vi "thermalImage_main02.vi"() -> ()   [LabVIEW 2018]
doc: "This example performs writes and reads on a serial port, as directed by the user. You can press the Write and Read buttons, and change the Read Count, while the example is running.\n\nThe parameters set for the serial port must match the parameters of the connected instrument or device. In this example, the Read Count parameter specifies the number of bytes that the serial port reads. If there were more bytes at the port than the specified number, those bytes would not be read. If there were less bytes at the port than the specified number, you would receive a timeout error.\n\nThis example expands upon the flow control options for XON and XOFF, allowing the user to choose those control characters. Also, the user can enable or disable a termination character. Some devices require a termination character in order to identify the end of command strings. Some devices send a termination character to signify the end of data to be read. This example shows how you can end the Read operation once a termination character is detected in the buffer and/or append a termination character at the end of the Write data."
uses:
  <vilib>/userdefined/High Color/IMAQdx.ctl
  <vilib>/Instr/_visa.llb/VISA Configure Serial Port (Instr).vi
  <vilib>/vision/driver/NI_Vision_Acquisition_Software.lvlib
  <vilib>/vision/NI_Vision_Development_Module.lvlib
panel:
  out "최대온도":dbl
  out "웨이브폼 차트":dbl(graph)
  in  "Frames Per Second":u32=10
  in  "AVI Path":path=path "E:/temp/b.avi"
  in  "stop 4":bool
  in  "stop 3":bool
  out "Cam  2":T1(plugin-control)
  in  "Camera":T2="cam1"
  in  "stop":bool
  in  "stop 2":bool
  in  "폭":dbl=10.0
  in  "중심":dbl=35.0
  out "Temperature":dbl[][](graph)
  in  "Stop":bool
  in  "VISA resource name":refnum<visa-resource-name>="COM6"
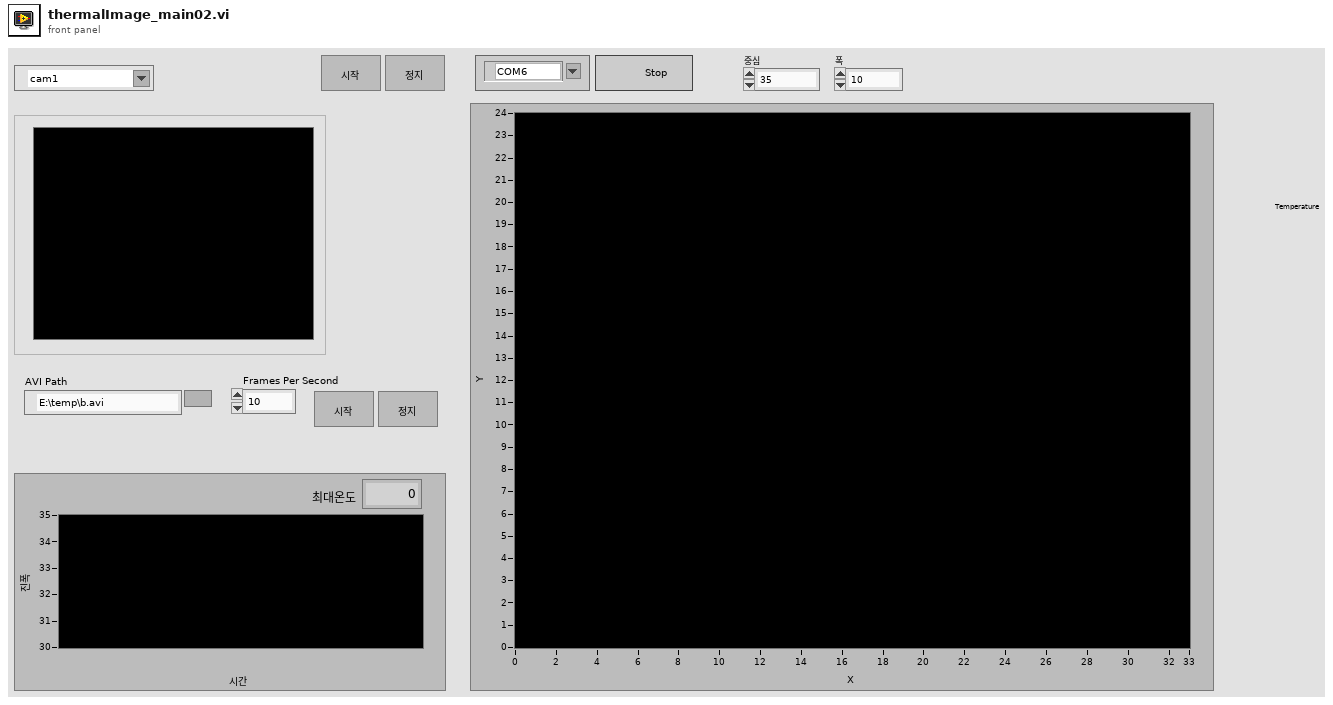
[diagram p1: front panel]
types:
  T1 = typedef "IMAQ Image.ctl" = refnum<image>
  T2 = typedef "IMAQdx.ctl" = refnum<k21>
  T3 = typedef "Image Type" = u32
  T4 = typedef "IMAQ AVI2 Refnum.ctl" = refnum<k20>
  T5 = typedef "imagedata.ctl" = cluster{"image type":i32, "image depth":i32, "image":u8[], "mask":u8[], "colors":u32[], "Rectangle":cluster{"left":i16, "top":i16, "right":i16, "bottom":i16}}
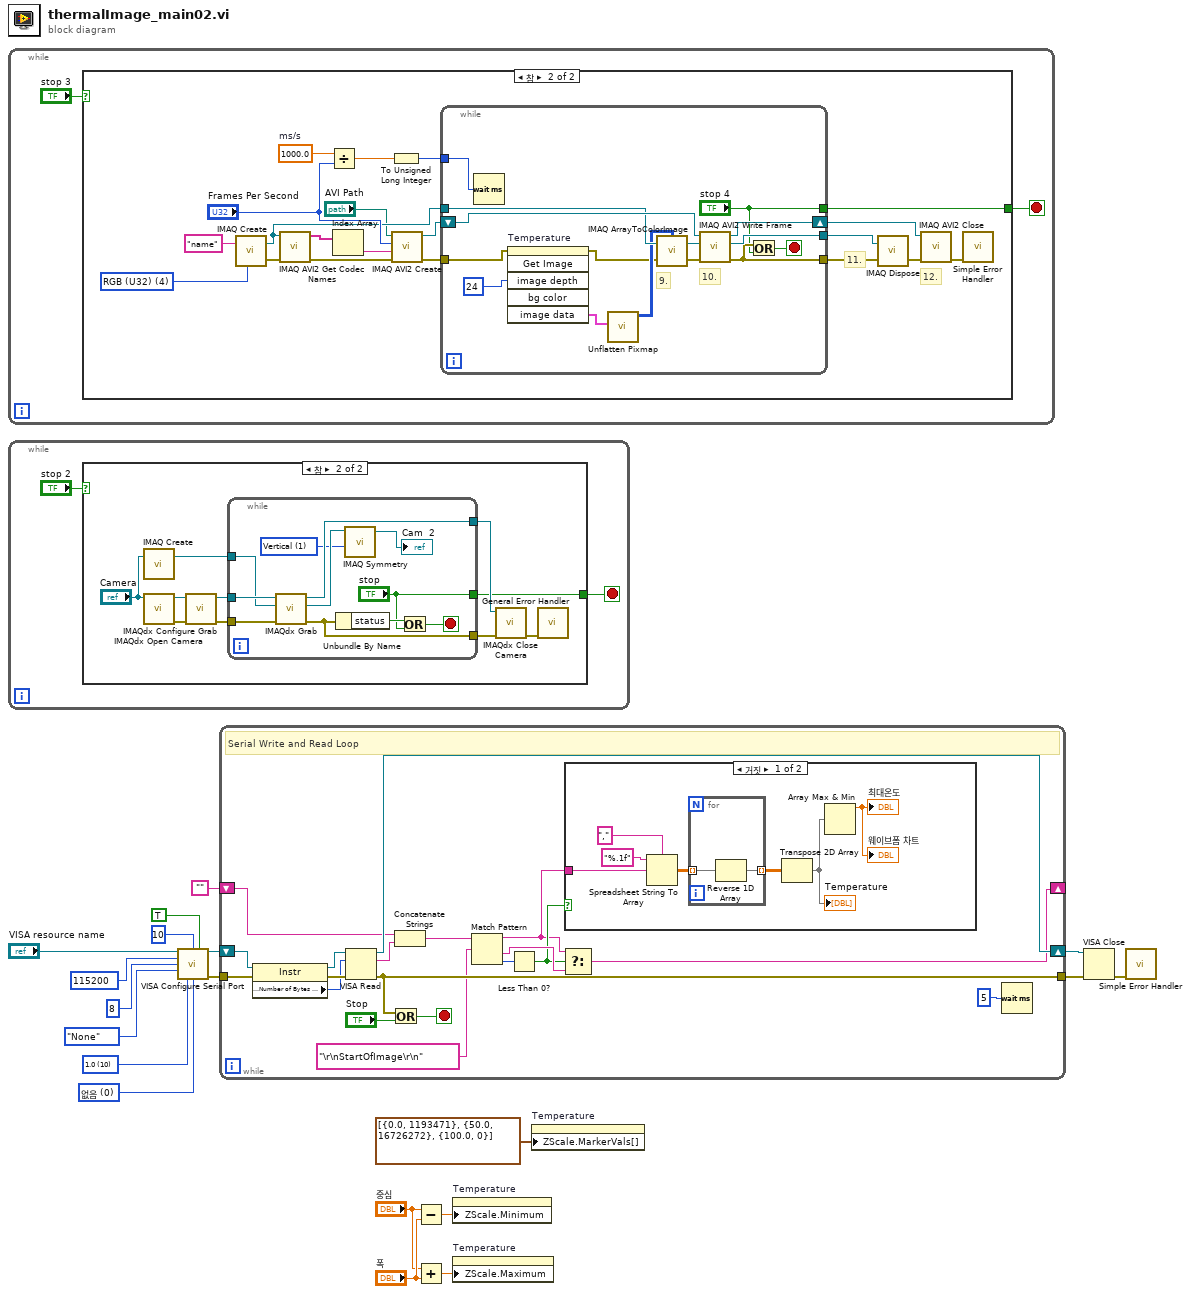
[diagram p0: block diagram]
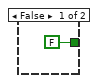
[diagram p2: hidden frame]
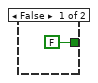
[diagram p3: hidden frame]
diagram:
  w6 = u16 0 items=["없음", "XON/XOFF", "RTS/CTS", "XON/XOFF & RTS/CTS", "DTR/DSR", "XON/XOFF & DTR/DSR"] ("flow control (0:none)")
  w7 = u16 10 items=["1.0"=10, "1.5"=15, "2.0"=20] ("stop bits (10: 1 bit)")
  n1 = while {
    stop <- w20 stop-if-true
    n2 = case shown="참" "stop 3" {
      tunnel: [FALSE ("stop") w23] -> w20
      frame False {
      }
      frame True {
        w26 = 1000.0  # ms/s
        w24 = T3 4 items=["Grayscale (U8)", "Grayscale (I16)", "Grayscale (SGL)", "Complex (CSG)", "RGB (U32)", "HSL (U32)", "RGB (U64)", "Grayscale (U16)"] ("Image Type")
        # "12."
        # "11."
        n3 = call "IMAQ Create"("Image Name"="name", "Image Type"=w24) -> ("New Image"=w36:T1, "error out"=w35:errorcluster)  [unwired: 3 in]
        n4 = call "IMAQ AVI2 Get Codec Names"("error in (no error)"=w35, "Image"=w36) -> ("error out"=w34:errorcluster, "Codec Names"=w38:string[])  [unwired: 8 in]
        n5 = Divide(x=w26, y="Frames Per Second") -> (x/y=w41:dbl)
        n6 = Index Array(array=w38) -> (element=w39:string)  [unwired: 1 in]
        n7 = To Unsigned Long Integer(number=w41) -> (unsigned 32bit integer=w42:u32)
        n8 = call "IMAQ AVI2 Create"("error in (no error)"=w34, "Codec"=w39, "Frames Per Second"="Frames Per Second", "AVI Path"="AVI Path") -> ("error out"=w37:errorcluster, "AVI Refnum"=w33:T4)  [unwired: 6 in]
        n9 = while {
          tunnel: w36 -> [w51]
          tunnel: w37 -> [w45]
          tunnel: [w55] -> w27
          tunnel: [w52] -> w28
          shift-right: [w56] -> w29
          shift-left: w33 -> [w57]
          tunnel: w42 -> [w54]
          tunnel: ["stop 4"] -> w23
          stop <- w53 stop-if-true
          # "10."
          # "9."
          n10 = Wait (ms)(milliseconds to wait=w54) -> ()  [unwired: 1 out]
          n11 = invoke on="Temperature" class="IntGraph (엄격한)" method="Get Image"(error in=w45, "image depth"=24 ("Image Depth")) -> (error out=w44:errorcluster, "image data"=w46:T5)  [unwired: 4 in, 4 out]
          n12 = call <vilib>:"Unflatten Pixmap.vi"("image data"=w46) -> ("24-bit pixmap"=w48:u32[][])  [unwired: 4 in, 6 out]
          n13 = call "IMAQ ArrayToColorImage"("Image Pixels (U32)"=w48, "Image"=w51, "error in (no error)"=w44) -> ("Image Out"=w50:T1, "error out"=w49:errorcluster)  [unwired: 2 in]
          n14 = call "IMAQ AVI2 Write Frame"("error in (no error)"=w49, "Image"=w50, "AVI Refnum"=w57) -> ("error out"=w52:errorcluster, "Image Out (duplicate)"=w55:T1, "AVI Refnum (duplicate)"=w56:T4)  [unwired: 6 in]
          n15 = Or(x=w52, y="stop 4") -> (x .or. y?=w53:bool)
        }
        n16 = call "IMAQ Dispose"("Image"=w27, "error in (no error)"=w28) -> ("error out"=w30:errorcluster)  [unwired: 4 in]
        n17 = call "IMAQ AVI2 Close"("error in (no error)"=w30, "AVI Refnum"=w29) -> ("error out"=w31:errorcluster)  [unwired: 9 in]
        n18 = call <vilib>:"Simple Error Handler.vi"("error in (no error)"=w31) -> ()  [unwired: 4 in, 5 out]
      }
    }
  }
  n19 = while {
    stop <- w58 stop-if-true
    n20 = case shown="참" "stop 2" {
      tunnel: [FALSE ("stop") w61] -> w58
      frame False {
      }
      frame True {
        n21 = call "IMAQ Create"("Image Name"="Camera") -> ("New Image"=w70:T1)  [unwired: 3 in, 2 out]
        n22 = call <vilib>:"IMAQdx Open Camera.vi"("Session In"="Camera") -> ("error out"=w64:errorcluster, "Session Out"=w66:T2)  [unwired: 2 in, 7 out]
        n23 = call <vilib>:"IMAQdx Configure Grab.vi"("error in"=w64, "Session In"=w66) -> ("error out"=w62:errorcluster, "Session Out"=w63:T2)  [unwired: 1 in, 7 out]
        n24 = while {
          tunnel: [w76] -> w69
          tunnel: w62 -> [w78]
          tunnel: w63 -> [w79]
          tunnel: [w75] -> w68
          tunnel: w70 -> [w77]
          tunnel: ["stop"] -> w61
          stop <- w81 stop-if-true
          w71 = u32 1 items=["Horizontal", "Vertical", "Central", "1st Diagonal", "2nd Diagonal"] ("Type of Symmetry")
          n25 = call <vilib>:"IMAQdx Grab.vi"("error in"=w78, "Image In"=w77, "Session In"=w79) -> ("error out"=w75:errorcluster, "Image Out"=w73:T1, "Session Out"=w76:T2)  [unwired: 5 in, 1 out]
          n26 = Unbundle By Name(w75) -> ("status"=w80:bool)
          n27 = call "IMAQ Symmetry"("Type of Symmetry"=w71, "Image Src"=w73) -> ("Image Dst Out"=→"Cam  2":T1)  [unwired: 3 in, 1 out]
          n28 = Or(x=w80, y="stop") -> (x .or. y?=w81:bool)
        }
        n29 = call <vilib>:"IMAQdx Close Camera.vi"("error in"=w68, "Session In"=w69) -> ("error out"=w67:errorcluster)  [unwired: 9 out]
        n30 = call <vilib>:"General Error Handler.vi"("error in (no error)"=w67) -> ()  [unwired: 2 in, 13 out]
      }
    }
  }
  n31 = call-poly "VISA Configure Serial Port"("VISA resource name"="VISA resource name", "termination char\n(0xA = '\\n' = LF)"=u8 10 ("Termination Character"), "Enable Termination\nChar (T)"=TRUE ("End Read on Termination Character?"), "baud rate (9600)"=u32 115200, "data bits (8)"=u16 8, "parity (0:none)"=enum16{"None", "Odd", "Even", "Mark", "Space"}."None", "stop bits (10: 1 bit)"=w7, "flow control (0:none)"=w6) -> ("VISA resource name out"=w13:refnum<visa-resource-name>, "error out"=w12:errorcluster)  [unwired: 2 in, 4 out]
  n32 = while {
    shift-right: [w95] -> w15
    shift-left: w13 -> [w97]
    tunnel: w12 -> [w93]
    tunnel: [w89] -> w16
    shift-right: [w82] -> _
    shift-left: "" -> [w91]
    stop <- w99 stop-if-true
    # "Serial Write and Read Loop"
    n33 = property class="Instr"(reference=w97, error in=w93) -> (reference out=w96:refnum<visa-resource-name>, error out=w94:errorcluster, "Serial Settings:Number of Bytes at Serial Port"=w92:u32)
    n34 = VISA Read(VISA resource name=w96, byte count=w92, error in (no error)=w94) -> (VISA resource name out=w95:refnum<visa-resource-name>, read buffer=w90:string, error out=w89:errorcluster)  [unwired: 1 out]
    n35 = Or(x=w89, y="Stop") -> (x .or. y?=w99:bool)
    n36 = Concatenate Strings(w91, w90) -> (w87:string)
    n37 = Match Pattern(string=w87, regular expression="\r\nStartOfImage\r\n") -> (before substring=w83:string, after substring=w85:string, offset past match=w86:i32)  [unwired: 1 in, 1 out]
    n38 = Less Than 0?(x=w86) -> (x < 0?=w84:bool)
    n39 = Select(t=w83, s=w84, f=w85) -> (s? t:f=w82:string)
    n40 = case shown="거짓" w84 {
      tunnel: w83 -> [w106 _]
      frame False {
        n41 = Spreadsheet String To Array(delimiter (Tab)=",", format string="%.1f", spreadsheet string=w106) -> (array=w104:dbl[][])  [unwired: 1 in]
        n42 = for {
          tunnel: w104 -> [w109] mode=indexing
          tunnel: [w108] -> w103 mode=indexing
          n43 = Reverse 1D Array(array=w109) -> (reversed array=w108:dbl[])
        }
        n44 = Transpose 2D Array(2D array=w103) -> (transposed array=w101:dbl[][])
        "Temperature" <- w101
        n45 = Array Max & Min(array=w101) -> (max value=→"최대온도" →"웨이브폼 차트":dbl)  [unwired: 3 out]
      }
      frame True {
      }
    }
    n46 = Wait (ms)(milliseconds to wait=u32 5) -> ()  [unwired: 1 out]
  }
  n47 = Subtract(x="중심", y="폭") -> (x-y=w5:dbl)
  n48 = Add(x="중심", y="폭") -> (x+y=w1:dbl)
  n49 = property on="Temperature" class="IntGraph (엄격한)"("ZScale.Minimum"=w5) -> ()  [unwired: 2 in, 2 out]
  n50 = property on="Temperature" class="IntGraph (엄격한)"("ZScale.Maximum"=w1) -> ()  [unwired: 2 in, 2 out]
  n51 = property on="Temperature" class="IntGraph (엄격한)"("ZScale.MarkerVals[]"=cluster{dbl, u32}[] [{0.0, 1193471}, {50.0, 16726272}, {100.0, 0}] ("Z 스케일.마커 값[]")) -> ()  [unwired: 2 in, 2 out]
  n52 = VISA Close(VISA resource name=w15, error in (no error)=w16) -> (error out=w17:errorcluster)
  n53 = call <vilib>:"Simple Error Handler.vi"("error in (no error)"=w17) -> ()  [unwired: 1 in, 8 out]
